vi "Drive Select.vi"(0 "Slow Turn":i32, 4 "Input 2 Y Axis":i32, 5 "Joystick 2":string="My Joystick RefNum", 6 "Input 2 X Axis":i32, 7 "Joystick 1":string="My Joystick RefNum", 8 "Input 1 Y Axis":i32, 9 "Input 1 X Axis":i32, 10 "Drive Train":string="RobotDrive", 11 "Mode":T1(ring)) -> (3 "Motor Values":dbl[](array[numeric]))   [LabVIEW 2015]
uses:
  <vilib>/Rock Robotics/WPI/Utilities/WPI_GetSetVariantRefNum.vi
  <vilib>/Rock Robotics/WPI/RobotDrive/WPI_RobotDriveArcadeDrive_Standard(NoSaturation).vi
panel:
  # "Drive Select\nby Chris Garuti\n\nModes: \nArcade:\nTakes X and Y from controller 1\n\nTank 1 Stick:\nX axis becomes left axis value and Y axis\n becomes right axis value from controller 1\n\nTank 2 Stick\nInput 1 Y axis becomes left axis value and Input 2 Y\n axis becomes right axis value\n\nCheesy Drive\nInput 1 Y axis becomes throttle and Input 2 X\naxis becomes turning. slow turn is on input 1"
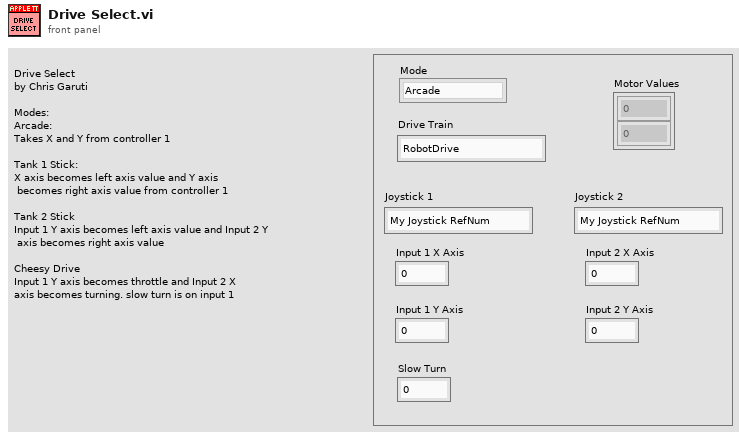
[diagram p1: front panel]
types:
  T1 = enum16{"Arcade", "Tank 1 Stick", "Tank 2 Stick", "Cheesey Drive"}
  T2 = typedef "WPI_RobotDriveDevRef.ctl" = cluster{"DevStatus":errorcluster, "Motors[]":T3[], "Square Inputs":bool, "Max Output":dbl}
  T3 = typedef "WPI_MotorControlDeviceRef.ctl" = cluster{"DeviceStatus":errorcluster, "Type":T4, "PWM":cluster{"PWM Channel":T5, "DeadBand":T6}, "CAN":cluster{"Device Number":u8, "Control Mode":T7, "Semaphore":T8, "Max Vout":dbl, "TalonSRX Control Mode":T9}, "Invert":bool}
  T4 = typedef "WPI_MotorControlType.ctl" = enum16{"PWM", "CAN", "CANTalonSRX"}
  T5 = typedef "FPGA_DIOPWMChannel.ctl" = enum8{"PWM 0", "PWM 1", "PWM 2", "PWM 3", "PWM 4", "PWM 5", "PWM 6", "PWM 7", "PWM 8", "PWM 9", "PWM MXP 0", "PWM MXP 1", "PWM MXP 2", "PWM MXP 3", "PWM MXP 4", "PWM MXP 5", "PWM MXP 6", "PWM MXP 7", "PWM MXP 8", "PWM MXP 9", "Invalid"}
  T6 = typedef "WPI_PWMDeadband.ctl" = cluster{"Name":string, "maxPositivePwm":i32, "minPositivePwm":i32, "centerPwm":i32, "maxNegativePwm":i32, "minNegativePwm":i32, "angularRange":u16}
  T7 = typedef "WPI_CANJaguar_ControlMode.ctl" = enum8{"Percent VBus", "Current", "Speed", "Position", "Voltage"}
  T8 = typedef "Semaphore RefNum" = refnum<k1>
  T9 = typedef "WPI_CANTalonSRX_APIControlMode.ctl" = enum8{"Percent VBus", "Speed", "Position", "Slave", "Unchanged / Invalid", "Voltage Compensation", "Current", "Motion Profile"}
  T10 = typedef "WPI_JoystickDevRef.ctl" = cluster{"Device":T11}
  T11 = typedef "WPI_JoystickDeviceEnum.ctl" = enum16{"USB 0", "USB 1", "USB 2", "USB 3", "USB 4", "USB 5"}
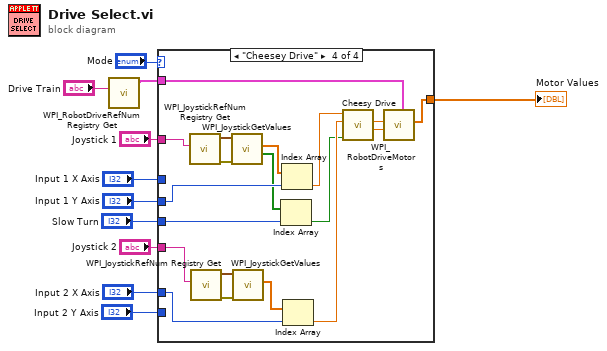
[diagram p0: block diagram]
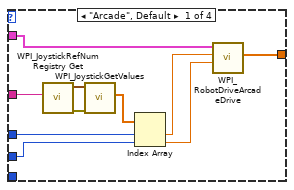
[diagram p2: hidden frame]
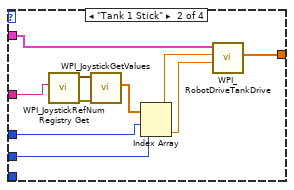
[diagram p3: hidden frame]
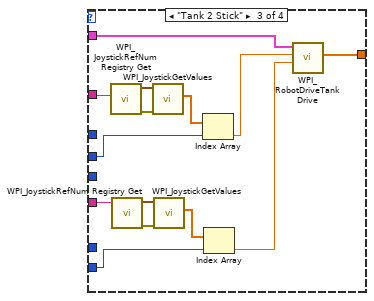
[diagram p4: hidden frame]
diagram:
  n1 = call <vilib>:"WPI_RobotDriveRefNum Registry Get.vi"("refnum name"="Drive Train") -> ("RobotDriveDevRef"=w8:T2)  [unwired: 9 in, 1 out]
  n2 = case shown="\"Cheesey Drive\"" "Mode" {
    tunnel: "Joystick 1" -> [w21 w26 w38 w58]
    tunnel: w8 -> [w13 w25 w32 w49]
    tunnel: "Input 1 X Axis" -> [w17 w23 _ _]
    tunnel: "Input 1 Y Axis" -> [w16 w22 w36 w56]
    tunnel: [w12 w24 w33 w48] -> w5
    tunnel: "Joystick 2" -> [_ _ w37 w57]
    tunnel: "Input 2 X Axis" -> [_ _ _ w55]
    tunnel: "Input 2 Y Axis" -> [_ _ w35 _]
    tunnel: "Slow Turn" -> [_ _ _ w46]
    frame "Arcade", Default {
      n3 = call <vilib>:"WPI_JoystickRefNum Registry Get.vi"("refnum name"=w21) -> ("error out"=w20:errorcluster, "JoystickDevRef"=w19:T10)  [unwired: 9 in]
      n4 = call <vilib>:"WPI_JoystickGetValues.vi"("error in (no error)"=w20, "JoystickDevRef"=w19) -> ("Axes"=w18:dbl[])  [unwired: 5 in, 4 out]
      n5 = Index Array(array=w18, index #1=w17, index #2=w16) -> (element #1=w15:dbl, element #2=w14:dbl)
      n6 = call-poly <vilib>:"WPI_RobotDriveArcadeDrive.vi"("Y axis value"=w14, "X axis value"=w15, "RobotDriveDevRef"=w13) -> ("Motor Values"=w12:dbl[])  [unwired: 6 in, 2 out]
    }
    frame "Tank 1 Stick" {
      n7 = call <vilib>:"WPI_JoystickRefNum Registry Get.vi"("refnum name"=w26) -> ("error out"=w31:errorcluster, "JoystickDevRef"=w30:T10)  [unwired: 9 in]
      n8 = call <vilib>:"WPI_JoystickGetValues.vi"("error in (no error)"=w31, "JoystickDevRef"=w30) -> ("Axes"=w29:dbl[])  [unwired: 5 in, 4 out]
      n9 = Index Array(array=w29, index #1=w23, index #2=w22) -> (element #1=w28:dbl, element #2=w27:dbl)
      n10 = call <vilib>:"WPI_RobotDriveTankDrive.vi"("Right axis value"=w27, "Left axis value"=w28, "RobotDriveDevRef"=w25) -> ("Motor Values"=w24:dbl[])  [unwired: 6 in, 2 out]
    }
    frame "Tank 2 Stick" {
      n11 = call <vilib>:"WPI_JoystickRefNum Registry Get.vi"("refnum name"=w38) -> ("error out"=w45:errorcluster, "JoystickDevRef"=w44:T10)  [unwired: 9 in]
      n12 = call <vilib>:"WPI_JoystickRefNum Registry Get.vi"("refnum name"=w37) -> ("error out"=w41:errorcluster, "JoystickDevRef"=w40:T10)  [unwired: 9 in]
      n13 = call <vilib>:"WPI_JoystickGetValues.vi"("error in (no error)"=w45, "JoystickDevRef"=w44) -> ("Axes"=w43:dbl[])  [unwired: 5 in, 4 out]
      n14 = call <vilib>:"WPI_JoystickGetValues.vi"("error in (no error)"=w41, "JoystickDevRef"=w40) -> ("Axes"=w39:dbl[])  [unwired: 5 in, 4 out]
      n15 = Index Array(array=w43, index=w36) -> (element=w42:dbl)
      n16 = Index Array(array=w39, index=w35) -> (element=w34:dbl)
      n17 = call <vilib>:"WPI_RobotDriveTankDrive.vi"("Right axis value"=w34, "Left axis value"=w42, "RobotDriveDevRef"=w32) -> ("Motor Values"=w33:dbl[])  [unwired: 6 in, 2 out]
    }
    frame "Cheesey Drive" {
      n18 = call <vilib>:"WPI_JoystickRefNum Registry Get.vi"("refnum name"=w58) -> ("error out"=w64:errorcluster, "JoystickDevRef"=w63:T10)  [unwired: 9 in]
      n19 = call <vilib>:"WPI_JoystickRefNum Registry Get.vi"("refnum name"=w57) -> ("error out"=w61:errorcluster, "JoystickDevRef"=w60:T10)  [unwired: 9 in]
      n20 = call <vilib>:"WPI_JoystickGetValues.vi"("error in (no error)"=w64, "JoystickDevRef"=w63) -> ("Buttons"=w52:bool[], "Axes"=w62:dbl[])  [unwired: 5 in, 3 out]
      n21 = call <vilib>:"WPI_JoystickGetValues.vi"("error in (no error)"=w61, "JoystickDevRef"=w60) -> ("Axes"=w59:dbl[])  [unwired: 5 in, 4 out]
      n22 = Index Array(array=w52, index=w46) -> (element=w47:bool)
      n23 = Index Array(array=w62, index=w56) -> (element=w54:dbl)
      n24 = Index Array(array=w59, index=w55) -> (element=w53:dbl)
      n25 = call "Cheesy Drive.vi"("Slow turn"=w47, "Turn"=w53, "Throttle"=w54) -> ("Right"=w51:dbl, "Left"=w50:dbl)  [unwired: 5 in]
      n26 = call <vilib>:"WPI_RobotDriveMotors.vi"("RightSpeed"=w51, "LeftSpeed"=w50, "RobotDriveDevRef"=w49) -> ("Motor Values"=w48:dbl[])  [unwired: 6 in, 2 out]
    }
  }
  "Motor Values" <- w5
